vi "Pre Launch Init.vi"(11 "Actor_Autotest in":refnum<class "Actor_Autotest.lvclass">) -> (0 "error out":errorcluster, 3 "Actor_Autotest out":refnum<class "Actor_Autotest.lvclass">)   [LabVIEW 2020, in "Library Core.lvlib" / "Actor_Autotest.lvlib" / "Actor_Autotest.lvclass"]
doc: "(<B>Filename</B>: Actor Framework.lvlib:Actor.lvclass:Pre Launch Init.vi)\n\nDefines behavior that occurs after the Launch Nested Actor method is invoked but before the actor's Actor Core method begins running.\n\nBy default, this method does nothing. A descendant class may override it to define behavior."
uses:
  Actor_Autotest.lvclass
  C:/Program Files (x86)/National Instruments/LabVIEW 2020/vi.lib/ActorFramework/Actor/Actor.lvclass
  <vilib>/ActorFramework/Actor/Actor.lvclass/Actor.ctl
  <vilib>/ActorFramework/Message Enqueuer/Message Enqueuer.lvclass/Message Enqueuer.ctl
  Actor_Autotest.lvclass/Actor_Autotest.ctl
  Instrument/Instrument (Default)/Class Instrument (Default).lvclass
  <vilib>/ActorFramework/Message Enqueuer/Init from Existing Queue.vi
  <vilib>/ActorFramework/Message Enqueuer/Message Enqueuer.lvclass
  <vilib>/ActorFramework/Actor/Actor.lvclass
  Commun VI/Library Commun.lvlib
panel:
  # "User Event created for stoping the actor core loop, and the name for the notifier"
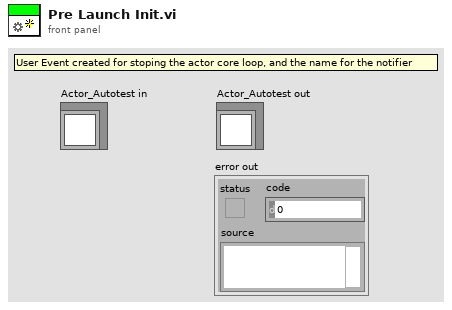
[diagram p1: front panel]
types:
  T1 = enum16{"Init", "Add Actor", "Delete Actor", "Get Actor Queue", "Get Log Actor Queue", "List all actors"}
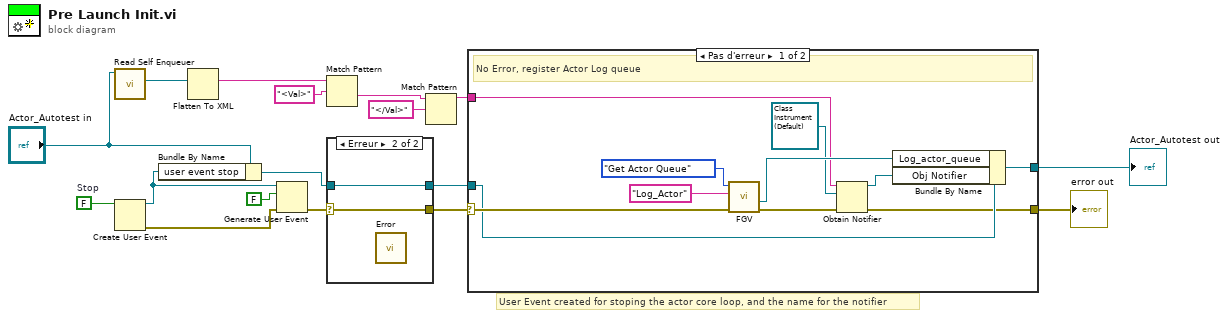
[diagram p0: block diagram]
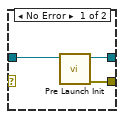
[diagram p2: hidden frame]
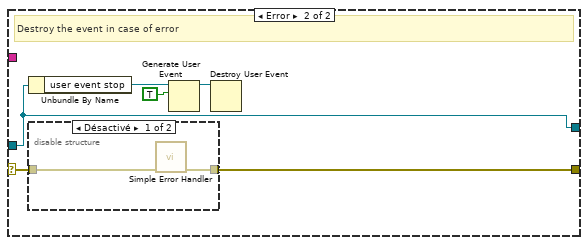
[diagram p3: hidden frame]
diagram:
  w17 = FALSE  # Stop
  # "User Event created for stoping the actor core loop, and the name for the notifier"
  n1 = call <vilib>:"Read Self Enqueuer.vi"("Actor"="Actor_Autotest in") -> ("Self Enqueuer"=w10:refnum<class "Message Enqueuer.lvclass">)  [unwired: 10 in]
  n2 = Create User Event(user event datatype=w17) -> (user event=w2:refnum<user-event>, error out=w3:errorcluster)  [unwired: 1 in]
  n3 = Bundle By Name(cluster="Actor_Autotest in", "user event stop"=w2) -> (w15:refnum<class "Actor_Autotest.lvclass">)
  n4 = Flatten To XML(6:w10) -> (2:w9:string)
  n5 = Generate User Event(user event=w2, event data cluster=FALSE ("event data"), error in=w3) -> (error out=w1:errorcluster)  [unwired: 1 in, 1 out]
  n6 = Match Pattern(string=w9, regular expression="<Val>") -> (after substring=w7:string)  [unwired: 1 in, 3 out]
  n7 = case shown="Erreur" w1 {
    selector: w1 -> [_ w22]
    tunnel: [w18 w22] -> w16
    tunnel: w15 -> [w20 w21]
    tunnel: [w19 w21] -> w14
    frame No Error {
      n8 = call-parent "Pre Launch Init.vi"("Actor in"=w20) -> ("error out"=w18:errorcluster, "Actor out"=w19:refnum<class "Actor_Autotest.lvclass">)  [unwired: 9 in]
    }
    frame Error {
      n9 = call "Error"() -> ()  [unwired: 10 in, 2 out]
    }
  }
  n10 = Match Pattern(string=w7, regular expression="</Val>") -> (before substring=w5:string)  [unwired: 1 in, 3 out]
  n11 = case shown="Pas d'erreur" w16 {
    selector: w16 -> [w32 w36]
    tunnel: w14 -> [w29 w35]
    tunnel: [w23 w34] -> w12
    tunnel: [w24 w35] -> w13
    tunnel: w5 -> [w27 _]
    frame No Error {
      # "No Error, register Actor Log queue"
      n12 = call "FGV.vi"("error in (no error)"=w32, "Actor name"="Log_Actor", "Action"=T1."Get Actor Queue") -> ("error out"=w31:errorcluster, "Actor's Queue Out"=w28:refnum<class "Message Enqueuer.lvclass">)  [unwired: 6 in, 1 out]
      n13 = Obtain Notifier(name (unnamed)=w27, notification data type=refnum<class "Class Instrument (Default).lvclass"> refnum ("notification"), error in (no error)=w31) -> (notifier out=w25:refnum<notifier>, error out=w23:errorcluster)  [unwired: 1 in, 1 out]
      n14 = Bundle By Name(cluster=w29, "Log_actor_queue"=w28, "Obj Notifier"=w25) -> (w24:refnum<class "Actor_Autotest.lvclass">)
    }
    frame Error {
      # "Destroy the event in case of error"
      n15 = Unbundle By Name(w35) -> ("user event stop"=w39:refnum<user-event>)
      n16 = disable-structure shown="Désactivé" {
        disable-tunnel: w36 -> [w41 _]
        disable-tunnel: [w40 _] -> w34
        frame Disabled {
          n17 = call <vilib>:"Simple Error Handler.vi"("error in (no error)"=w41) -> ("error out"=w40:errorcluster)  [unwired: 4 in, 4 out]
        }
        frame Enabled {
        }
      }
      n18 = Generate User Event(user event=w39, event data cluster=TRUE ("event data")) -> (user event out=w37:refnum<user-event>)  [unwired: 2 in, 1 out]
      n19 = Destroy User Event(user event=w37) -> ()  [unwired: 1 in, 1 out]
    }
  }
  "error out" <- w12
  "Actor_Autotest out" <- w13
